vi "Close.vi"(8 "error in (no error)":errorcluster, 11 "Logging in":refnum<class "Logging.lvclass">) -> (0 "error out":errorcluster)   [LabVIEW 2020, in "Logging.lvclass"]
uses:
  Logging.lvclass
  Logging.lvclass/Logging.ctl
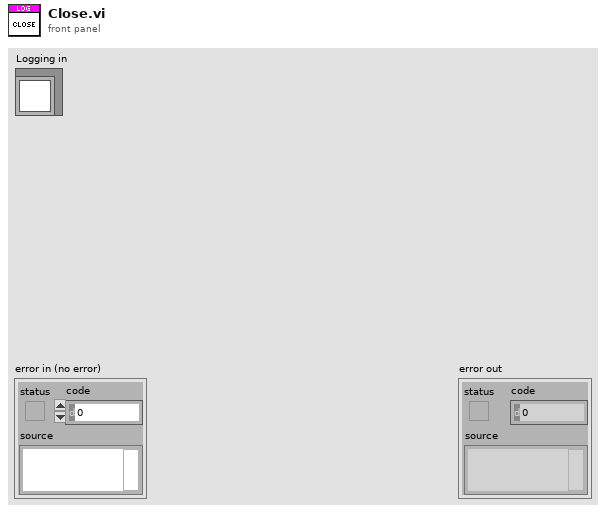
[diagram p1: front panel]
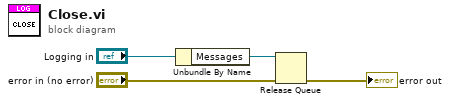
[diagram p0: block diagram]
diagram:
  n1 = Unbundle By Name("Logging in") -> ("Messages"=w1:refnum<queue>)
  n2 = Release Queue(queue=w1, error in (no error)="error in (no error)") -> (error out=→"error out":errorcluster)  [unwired: 1 in, 2 out]
